vi "generate sub-block test.vi"(8 "error in (no error)":errorcluster, 11 "Tdms File":refnum<k34>) -> (0 "error out":errorcluster, 3 "Tdms File Out":refnum<k34>)   [LabVIEW 2020]
doc: "Writes alternating segments of 2 sets of channels in the same group. ch1-3 at 1000 per write and 4-6 at 500 per write.\n\nEach pair of writes is alternated between interleaved and decimated data."
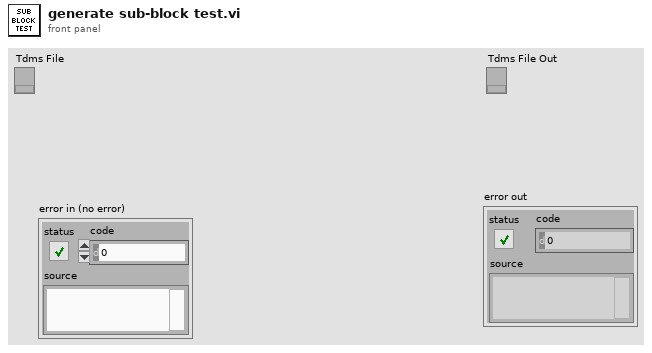
[diagram p1: front panel]
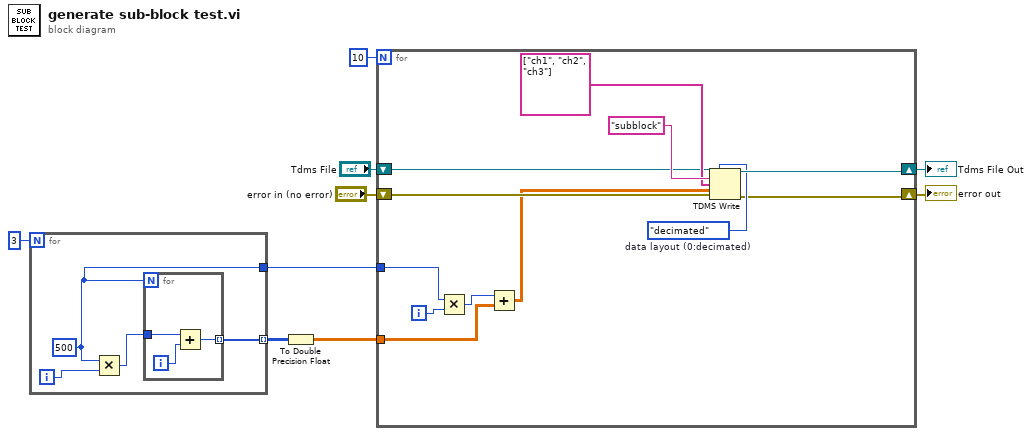
[diagram p0: block diagram]
diagram:
  n1 = for {
    N: 3 -> [_]
    tunnel: [w11] -> w8 mode=indexing
    tunnel: [w10] -> w1
    i -> [w13]
    w10 = 500 ("x")
    n2 = Multiply(x=w10, y=w13) -> (x*y=w12:i32)
    n3 = for {
      N: w10 -> [_]
      tunnel: w12 -> [w15]
      tunnel: [w14] -> w11 mode=indexing
      i -> [w16]
      n4 = Add(x=w15, y=w16) -> (x+y=w14:i32)
    }
  }
  n5 = To Double Precision Float(number=w8) -> (double precision float=w6:dbl[][])
  n6 = for {
    N: 10 -> [_]
    tunnel: w6 -> [w21]
    shift-right: [w25] -> w4
    shift-left: "Tdms File" -> [w26]
    shift-right: [w23] -> w2
    shift-left: "error in (no error)" -> [w22]
    tunnel: w1 -> [w19]
    i -> [w20]
    w24 = enum16{"decimated", "interleaved"}."decimated"  # data layout (0:decimated)
    n7 = Multiply(x=w19, y=w20) -> (x*y=w18:i32)
    n8 = Add(x=w18, y=w21) -> (x+y=w17:dbl[][])
    n9 = TDMS Write(0:w26, 1:w24, 5:"subblock" ("group name in (Untitled)"), 7:string[] ["ch1", "ch2", "ch3"] ("channel name(s) in (Untitled)"), 9:w17, 11:w22) -> (4:w25:refnum<k34>, 15:w23:errorcluster)  [unwired: 2 out]
  }
  "Tdms File Out" <- w4
  "error out" <- w2
